vi "Add Subscriber.vi"(8 "error in (no error)":errorcluster, 10 "New FIFO Instance Config":T1, 11 "CIF_Fifo_U8 in":refnum<class "CIF_Fifo_U8_Multi.lvclass">) -> (0 "error out":errorcluster, 2 "New Publisher":string, 3 "CIF_Fifo_U8 out":refnum<class "CIF_Fifo_U8_Multi.lvclass">)   [LabVIEW 2021, in "CIF_Fifo_U8_Multi.lvclass"]
uses:
  CIF_Fifo_U8_Multi.lvclass
  D:/dev/Packages/Channel_Manager/src/CIFChannels/CIFChannels.lvclass
  ChannelCommon/typedef/New FIFO Instance Configuration.ctl
  CIF_Fifo_U8_Multi.lvclass/CIF_Fifo_U8_Multi.ctl
  CIFChannels/Typedef/Direction.ctl
  FIFO_U8/CIF_NIChn_Fifo_U8.lvclass
  CIFChannels/CIFChannels.lvclass
  ChannelCommon/ChannelCommon.lvlib
  D:/dev/Packages/Channel_Manager/src/CIF_NIChn/FIFO_U8/CIF_NIChn_Fifo_U8.lvclass
  D:/dev/Packages/Channel_Manager/src/CIF_NIChn/NIChn/CIF_NIChn.lvclass
  D:/dev/Packages/Channel_Manager/src/CIF_NIChn/FIFO_U8_Multi/CIF_Fifo_U8_Multi.lvclass
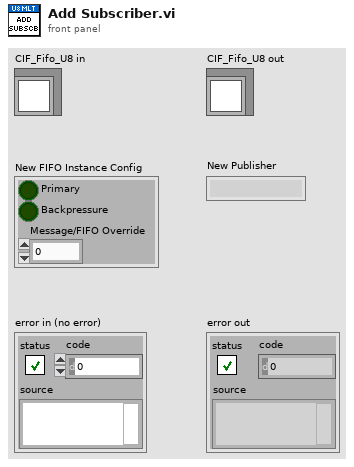
[diagram p1: front panel]
types:
  T1 = typedef "ChannelCommon.lvlib/New FIFO Instance Configuration.ctl" = cluster{"Primary":bool, "Backpressure":bool, "Message/FIFO Override":u32}
  T2 = typedef "CIFChannels.lvclass/Direction.ctl" = enum16{"Publisher", "Subscriber"}
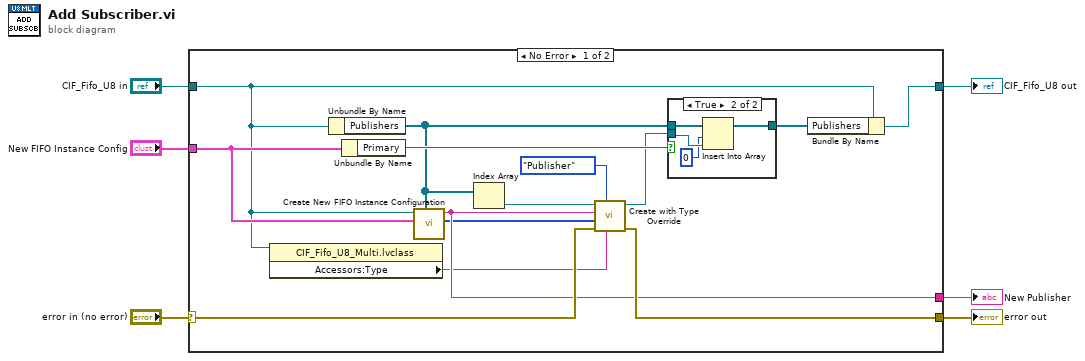
[diagram p0: block diagram]
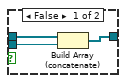
[diagram p2: hidden frame]
diagram:
  n1 = case shown="No Error" "error in (no error)" {
    selector: "error in (no error)" -> [w12 w29]
    tunnel: [w14 w29] -> w5
    tunnel: [w16 w28] -> w3
    tunnel: "CIF_Fifo_U8 in" -> [w8 w28]
    tunnel: "New FIFO Instance Config" -> [w13 _]
    tunnel: [w11 _] -> w1
    frame No Error {
      n2 = property class="CIF_Fifo_U8_Multi.lvclass"(reference=w8) -> ("Accessors:Type"=w7:string)  [unwired: 1 in, 2 out]
      n3 = Unbundle By Name(w8) -> ("Publishers"=w9:refnum<class "CIF_NIChn_Fifo_U8.lvclass">[])
      n4 = Unbundle By Name(w13) -> ("Primary"=w18:bool)
      n5 = call "Create New FIFO Instance Configuration.vi"("Publisher Array in"=w9, "New FIFO Instance Config"=w13, "CIFChannels.lvclass"=w8) -> ("Flattened FIFO Config"=w10:u8[], "New Publisher"=w11:string)  [unwired: 7 in]
      n6 = Index Array(array=w9) -> (element=w20:refnum<class "CIF_NIChn_Fifo_U8.lvclass">)  [unwired: 1 in]
      n7 = call "Create with Type Override.vi"("Type Override"=w7, "Direction"=Direction."Publisher", "error in (no error)"=w12, "Custom Config Data"=w10, "Name"=w11, "CIFFIFO in"=w20) -> ("error out"=w14:errorcluster, "CIFFIFO out"=w15:refnum<class "CIF_NIChn_Fifo_U8.lvclass">)  [unwired: 4 in]
      n8 = case shown="True" w18 {
        tunnel: w9 -> [w23 w27]
        tunnel: [w22 w24] -> w17
        tunnel: w15 -> [w21 w26]
        frame False {
          n9 = Build Array (concatenate)(w23, w21) -> (w22:refnum<class "CIF_NIChn_Fifo_U8.lvclass">[])
        }
        frame True {
          n10 = Insert Into Array(array=w27, index=0, new element=w26) -> (w24:refnum<class "CIF_NIChn_Fifo_U8.lvclass">[])
        }
      }
      n11 = Bundle By Name(cluster=w8, "Publishers"=w17) -> (w16:refnum<class "CIF_Fifo_U8_Multi.lvclass">)
    }
    frame Error {
    }
  }
  "error out" <- w5
  "CIF_Fifo_U8 out" <- w3
  "New Publisher" <- w1
